vi "Replay Example.vi"(6 "Trajectory Configuration":path=path "replay.json") -> (0 "error out":errorcluster, 1 "Number of frames":i32, 2 "fps":dbl, 3 "Camera":picture)   [LabVIEW 2019]
doc: "This example shows how to run the Simx client to configure the simulator on Replay mode."
uses:
  tools/simx_common.vi
  Lib_Simx.lvlib
panel:
  out "Current frame":i32
  out "Trajectory":string
  in  "stop":bool
  out "Weather Profiles":T1(array[cluster])
  # "Trajectory Configuration"
  # "Trajectory"
  # "FPS"
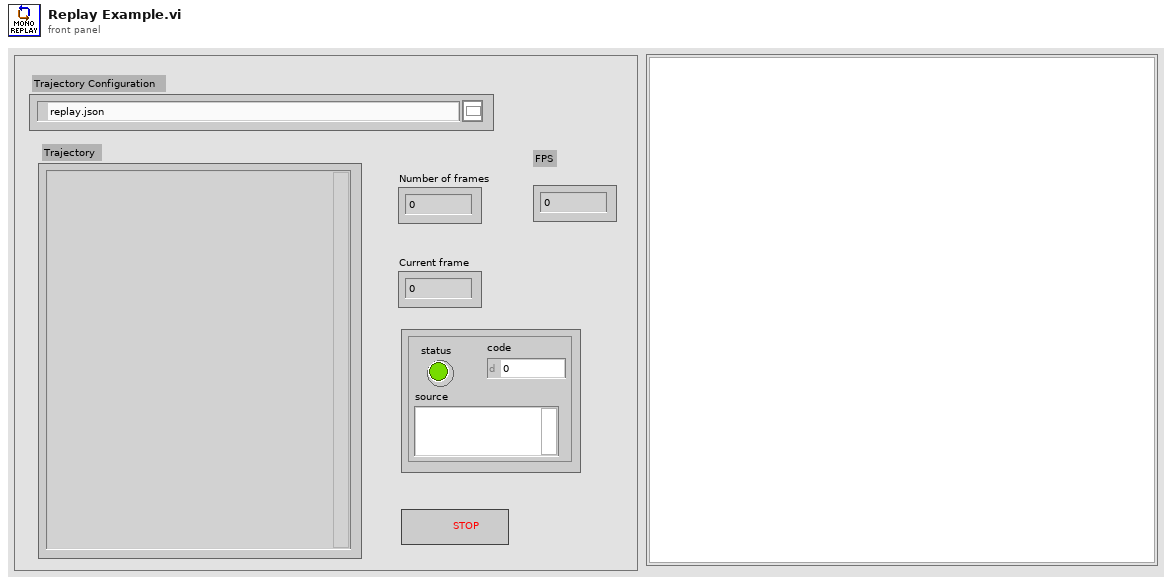
[diagram p1: front panel]
types:
  T1 = cluster{"id":string, "CloudColor":cluster{"A":sgl, "B":sgl, "G":sgl, "R":sgl}, "CloudOpacity":sgl, "Day":sgl, "FogCutoffDistance":sgl, "FogDensity":sgl, "FogHeightFalloff":sgl, "FogInscatteringColor":cluster{"A":sgl, "B":sgl, "G":sgl, "R":sgl}, "FogMaxOpacity":sgl, "FogStartDistance":sgl, "HorizonColor":cluster{"A":sgl, "B":sgl, "G":sgl, "R":sgl}, "HorizonFalloff":sgl, "Hours":sgl, "IsDaylightSavingTime":bool, "Latitude":sgl, "Longitude":sgl, "Minutes":sgl, "Month":sgl, "NorthOffset":sgl, "OverallSkyColor":cluster{"A":sgl, "B":sgl, "G":sgl, "R":sgl}, "OverideTimeBasedSunAngle":bool, "PrecipitationAccumulation":sgl, "PrecipitationAmount":sgl, "PrecipitationType":string, "SecondFogDensity":sgl, "SecondFogHeightFalloff":sgl, "SecondFogHeightOffset":sgl, "Seconds":sgl, "SkyLightColor":cluster{"A":sgl, "B":sgl, "G":sgl, "R":sgl}, "SkyLightIntensity":sgl, "StarBrightness":sgl, "SunAzimuthAngle":sgl, "SunBrightness":sgl, "SunDirectionalLightColor":cluster{"A":sgl, "B":sgl, "G":sgl, "R":sgl}, "SunDirectionalLightIntensity":sgl, "SunPolarAngle":sgl, "TimeZone":sgl, "WindAngle":sgl, "WindIntensity":sgl, "Year":sgl, "ZenithColor":cluster{"A":sgl, "B":sgl, "G":sgl, "R":sgl}, "bPrecipitation":bool, "bWind":bool}[]
  T2 = typedef "Lib_Simx.lvlib/simx_connection.ctl" = cluster{"Config":T3, "Connections":T6, "Map":cluster{"lanes":cluster{"x":dbl[], "y":dbl[], "z":dbl[]}, "StartPosition":cluster{"start_points":T7, "StartRotation":dbl[], "StartLocation":dbl[]}, "Draw Map Size":T8, "DrawArea":cluster{"min_Y":dbl, "min_X":dbl, "Scale X":dbl, "Scale Y":dbl}, "Map":picture, "Map Geojson":string}}
  T3 = typedef "Lib_Simx.lvlib/config.ctl" = cluster{"Trajectory":T4, "Weather":T5}
  T4 = typedef "Lib_Simx.lvlib/trajectory.ctl" = cluster{"Number of frames":i32, "Frame number":i32, "Trajectory":string}
  T5 = typedef "Lib_Simx.lvlib/weather.ctl" = cluster{"id":string}
  T6 = typedef "Lib_Simx.lvlib/connections.ctl" = cluster{"Simulator Connection":refnum<k5>, "server_ip":string, "Port":i32, "Sensor connections":refnum<k5>[]}
  T7 = typedef "Lib_Simx.lvlib/start_points.ctl" = cluster{"locations":dbl[][], "rotations":dbl[][], "type":string[]}
  T8 = typedef "LVBoundsTypeDef.ctl" = cluster{"Width":u32, "Height":u32}
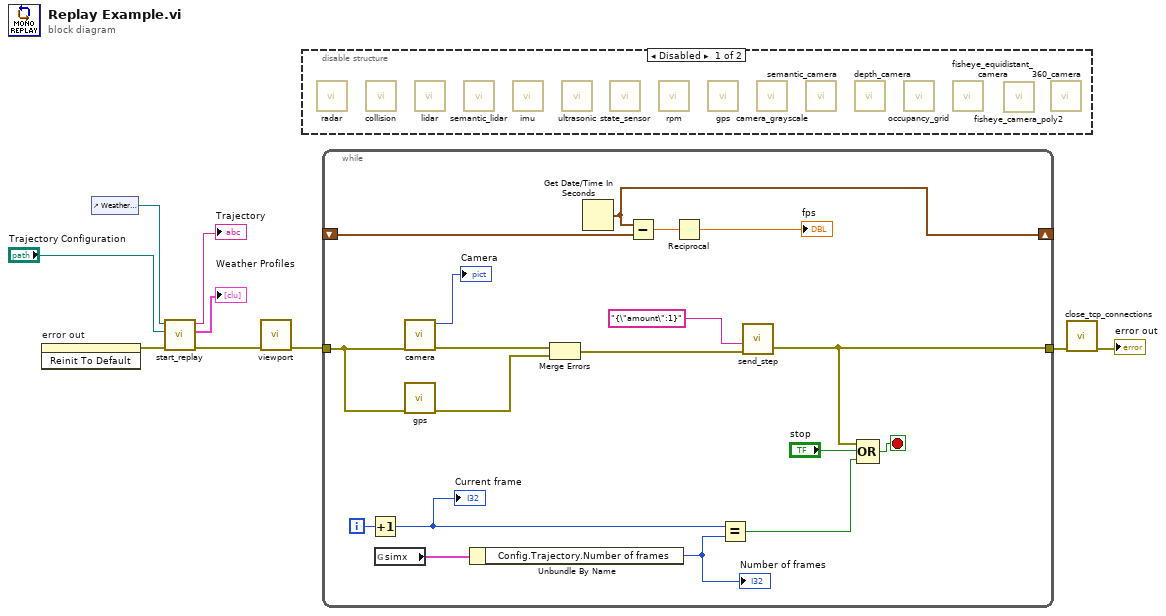
[diagram p0: block diagram]
diagram:
  n1 = invoke on="error out" class="Clust (strict)" method="Reinit To Default"() -> (error out=w4:errorcluster)  [unwired: 3 in, 2 out]
  n2 = control-ref of="Weather Profiles"() -> (w6:refnum<vi>)
  n3 = call "start_replay.vi"("error in"=w4, "Trajectory Configuration"="Trajectory Configuration", "Weather Ref"=w6) -> ("error out"=w2:errorcluster, "Weather Profiles"=→"Weather Profiles":T1, "Trajectory configuration"=→"Trajectory":string)  [unwired: 2 in]
  n4 = call "viewport.vi"("Error In"=w2) -> ("Error Out"=w3:errorcluster)  [unwired: 6 in]
  n5 = disable-structure shown="Disabled" {
    frame Disabled {
      n6 = call "radar.vi"() -> ()  [unwired: 4 in, 5 out]
      n7 = call "collision.vi"() -> ()  [unwired: 4 in, 4 out]
      n8 = call "lidar.vi"() -> ()  [unwired: 4 in, 4 out]
      n9 = call "semantic_lidar.vi"() -> ()  [unwired: 4 in, 4 out]
      n10 = call "imu.vi"() -> ()  [unwired: 4 in, 4 out]
      n11 = call "ultrasonic.vi"() -> ()  [unwired: 3 in, 4 out]
      n12 = call "state_sensor.vi"() -> ()  [unwired: 4 in, 4 out]
      n13 = call "rpm.vi"() -> ()  [unwired: 4 in, 4 out]
      n14 = call "gps.vi"() -> ()  [unwired: 4 in, 4 out]
      n15 = call "camera_grayscale.vi"() -> ()  [unwired: 5 in, 5 out]
      n16 = call "semantic_camera.vi"() -> ()  [unwired: 5 in, 5 out]
      n17 = call "depth_camera.vi"() -> ()  [unwired: 5 in, 5 out]
      n18 = call "occupancy_grid.vi"() -> ()  [unwired: 5 in, 5 out]
      n19 = call "fisheye_equidistant_camera.vi"() -> ()  [unwired: 5 in, 4 out]
      n20 = call "fisheye_camera_poly2.vi"() -> ()  [unwired: 5 in, 4 out]
      n21 = call "360_camera.vi"() -> ()  [unwired: 5 in, 4 out]
    }
    frame Enabled {
    }
  }
  n22 = while {
    shift-right: [w27] -> _
    shift-left: _ -> [w26]
    tunnel: w3 -> [w15]
    tunnel: [w21] -> w9
    i -> [w12]
    stop <- w23 stop-if-true
    n23 = Increment(x=w12) -> (x+1=w20:i32)
    "Current frame" <- w20
    n24 = global read "simx_common.vi" "simx"() -> (w14:T2)
    n25 = call "camera.vi"("error In"=w15) -> ("Image"=→"Camera":picture, "error out"=w11:errorcluster)  [unwired: 4 in, 3 out]
    n26 = call "gps.vi"("error in"=w15) -> ("error out"=w24:errorcluster)  [unwired: 3 in, 3 out]
    n27 = Unbundle By Name(w14) -> ("Config.Trajectory.Number of frames"=w19:i32)
    "Number of frames" <- w19
    n28 = Merge Errors(w11, w24) -> (w22:errorcluster)
    n29 = Get Date/Time In Seconds() -> (seconds since 1Jan1904=w27:timestamp)
    n30 = Subtract(x=w27, y=w26) -> (x-y=w25:dbl)
    n31 = Reciprocal(x=w25) -> (1/x=→"fps":dbl)
    n32 = Equal?(x=w20, y=w19) -> (x = y?=w18:bool)
    n33 = call "send_step.vi"("error in"=w22, "message"="{\"amount\":1}") -> ("error out"=w21:errorcluster)  [unwired: 3 in]
    n34 = Compound Arithmetic op=OR(w21, "stop", w18) -> (w23:bool)
  }
  n35 = call "close_tcp_connections.vi"("error in"=w9) -> ("error out"=→"error out":errorcluster)  [unwired: 6 in]
